vi "Update Boolean.vi"(8 "error in (no error)":errorcluster, 10 "Boolean":bool, 11 "Example Source in":refnum<class "Example Source.lvclass">) -> (0 "error out":errorcluster, 3 "Example Source out":refnum<class "Example Source.lvclass">)   [LabVIEW 2016, in "Example Source.lvlib" / "Example Source.lvclass"]
uses:
  Example Source.lvclass
  Example Source.lvclass/Example Source.ctl
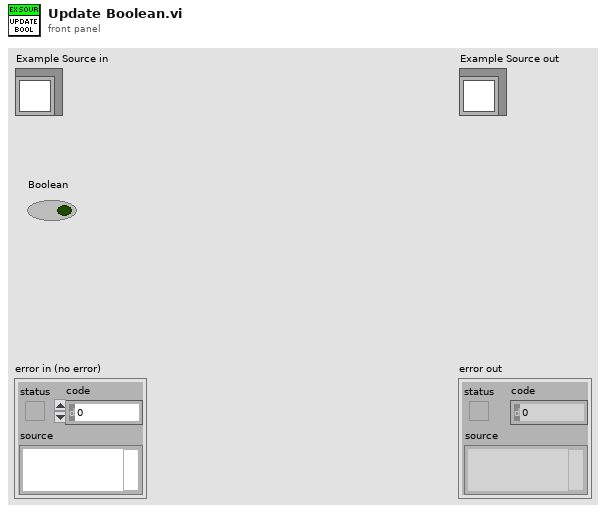
[diagram p1: front panel]
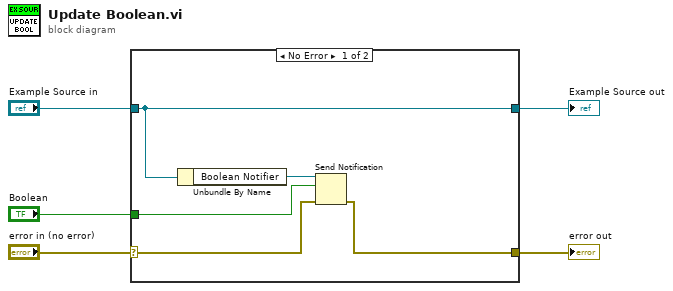
[diagram p0: block diagram]
diagram:
  n1 = case shown="No Error" "error in (no error)" {
    selector: "error in (no error)" -> [w8 w12]
    tunnel: [w7 w12] -> w4
    tunnel: [w10 w11] -> w2
    tunnel: "Example Source in" -> [w10 w11]
    tunnel: "Boolean" -> [w6 _]
    frame No Error {
      n2 = Unbundle By Name(w10) -> ("Boolean Notifier"=w9:refnum<notifier>)
      n3 = Send Notification(notification=w6, notifier=w9, error in (no error)=w8) -> (error out=w7:errorcluster)  [unwired: 1 out]
    }
    frame Error {
    }
  }
  "error out" <- w4
  "Example Source out" <- w2
